vi "Test Clear Snapshot.vi"() -> (0 "error out":errorcluster)   [LabVIEW 2020]
doc: "Test Clearing Snapshot Entry of a single VI."
uses:
  <vilib>/addons/_JKI Toolkits/Caraya/classes/Test/Test.lvclass
  src/Public API.lvlib
  src/Path Getter Mock/Path Getter Mock.lvclass
  src/Type Definitions/Snapshot Handling Options--cluster.ctl
  C:/Users/juanj/Documents/hasbun_wood_engineering/github/Debug-Snapshots-for-LabVIEW/src/Path Getter Mock/Path Getter Mock.lvclass
  C:/Users/juanj/Documents/hasbun_wood_engineering/github/Debug-Snapshots-for-LabVIEW/src/IPath Getter/IPath Getter.lvclass
  <vilib>/Utility/miscctls.llb/LVBreakpointStatusEnum.ctl
  src/Type Definitions/Class Name--enum.ctl
  src/Type Definitions/Breakpoint--cluster.ctl
  src/Type Definitions/Debug Snapshot--cluster.ctl
  src/Type Definitions/Debug Snapshot Array--cluster.ctl
  <vilib>/addons/_JKI Toolkits/Caraya/classes/Assert/Assert.lvclass
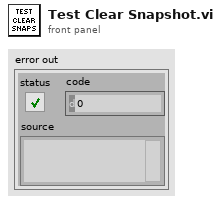
[diagram p1: front panel]
types:
  T1 = typedef "Debug Snapshot Array--cluster.ctl" = cluster{"Debug Snapshots":T2[]}
  T2 = typedef "Debug Snapshot--cluster.ctl" = cluster{"VI Name":string, "Breakpoints":T3[], "Probes":i32[]}
  T3 = typedef "Breakpoint--cluster.ctl" = cluster{"UID":i32, "BP Status":T4, "Class Name":T5}
  T4 = typedef "LVBreakpointStatusEnum.ctl" = enum8{"Cleared Break", "Enabled Break", "Disabled Break"}
  T5 = typedef "Class Name--enum.ctl" = enum16{"Node", "Wire"}
  T6 = typedef "Snapshot Handling Options--cluster.ctl" = cluster{"Breakpoints":bool, "Probes":bool}
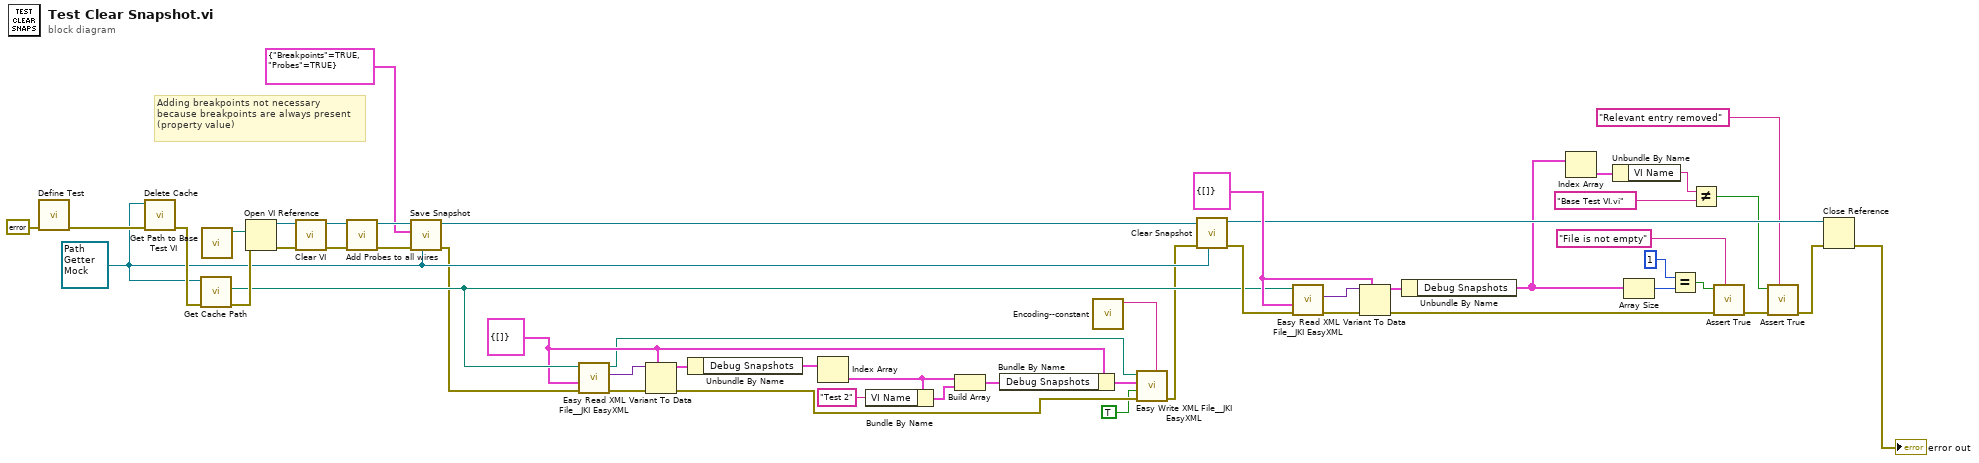
[diagram p0: block diagram]
diagram:
  w23 = T1 {"Debug Snapshots"=[]} ("Debug Snapshot Array")
  w37 = T1 {"Debug Snapshots"=[]} ("Debug Snapshot Array")
  w40 = refnum<class "Path Getter Mock.lvclass"> refnum ("Path Getter Mock.lvclass")
  # "Adding breakpoints not necessary\nbecause breakpoints are always present\n(property value)"
  n1 = call <vilib>:"Define Test.vi"("error in (no error)"=errorcluster {"status"=FALSE, "code"=0, "source"=""}) -> ("error out"=w49:errorcluster)  [unwired: 9 in, 1 out]
  n2 = call "Delete Cache.vi"("error in"=w49, "IPath Getter.lvclass"=w40) -> ("error out"=w46:errorcluster)  [unwired: 9 in]
  n3 = call-dynamic "Get Cache Path.vi"("error in"=w46, "Path Getter Mock in"=w40) -> ("error out"=w45:errorcluster, "Path"=w29:path)  [unwired: 8 in]
  n4 = call "Get Path to Base Test VI.vi"() -> ("Path"=w47:path)  [unwired: 11 in]
  n5 = Open VI Reference(vi path=w47, error in (no error)=w45) -> (vi reference=w2:refnum<vi>, error out=w48:errorcluster)  [unwired: 4 in]
  n6 = call "Clear VI.vi"("error in"=w48, "VI Refnum In"=w2) -> ("error out"=w3:errorcluster, "VI Refnum Out"=w1:refnum<vi>)  [unwired: 8 in]
  n7 = call "Add Probes to all wires.vi"("error in"=w3, "VI Refnum In"=w1) -> ("error out"=w43:errorcluster, "VI Refnum Out"=w44:refnum<vi>)  [unwired: 8 in]
  n8 = call "Save Snapshot.vi"("IPath Getter in"=w40, "error in"=w43, "Debug Elements Options"=T6 {"Breakpoints"=TRUE, "Probes"=TRUE}, "VI Reference in"=w44) -> ("error out"=w28:errorcluster, "VI Reference out"=w41:refnum<vi>)  [unwired: 6 in]
  n9 = call <vilib>:"Easy Read XML File__JKI EasyXML.vi"("error in (no error)"=w28, "LabVIEW Data (Type)"=w23, "XML File Path"=w29) -> ("error out"=w31:errorcluster, "LabVIEW Data"=w32:variant, "XML File Path (duplicate)"=w20:path)  [unwired: 6 in]
  n10 = Variant To Data(error in=w31, type=w23, Variant=w32) -> (data=w30:T1, error out=w19:errorcluster)
  n11 = Unbundle By Name(w30) -> ("Debug Snapshots"=w27:T2[])
  n12 = Index Array(array=w27) -> (element=w24:T2)  [unwired: 1 in]
  n13 = Bundle By Name(cluster=w24, "VI Name"="Test 2") -> (w25:T2)
  n14 = Build Array(w24, w25) -> (w22:T2[])
  n15 = Bundle By Name(cluster=w23, "Debug Snapshots"=w22) -> (w21:T1)
  n16 = call "Encoding--constant.vi"() -> ("Encoding (none)"=w18:string)  [unwired: 11 in]
  n17 = call <vilib>:"Easy Write XML File__JKI EasyXML.vi"("Encoding (none)"=w18, "error in (no error)"=w19, "Overwrite File? (false)"=TRUE, "LabVIEW Data"=w21, "XML File Path"=w20) -> ("error out"=w17:errorcluster)  [unwired: 5 in, 1 out]
  n18 = call "Clear Snapshot.vi"("IPath Getter.lvclass"=w40, "error in"=w17, "VI Reference in"=w41) -> ("error out"=w39:errorcluster, "VI Reference out"=w35:refnum<vi>)  [unwired: 7 in]
  n19 = call <vilib>:"Easy Read XML File__JKI EasyXML.vi"("error in (no error)"=w39, "LabVIEW Data (Type)"=w37, "XML File Path"=w29) -> ("error out"=w36:errorcluster, "LabVIEW Data"=w38:variant)  [unwired: 6 in, 1 out]
  n20 = Variant To Data(error in=w36, type=w37, Variant=w38) -> (data=w33:T1, error out=w34:errorcluster)
  n21 = Unbundle By Name(w33) -> ("Debug Snapshots"=w9:T2[])
  n22 = Index Array(array=w9) -> (element=w8:T2)  [unwired: 1 in]
  n23 = Unbundle By Name(w8) -> ("VI Name"=w10:string)
  n24 = Array Size(array=w9) -> (size(s)=w15:i32)
  n25 = Equal?(x=1, y=w15) -> (x = y?=w13:bool)
  n26 = Not Equal?(x=w10, y="Base Test VI.vi") -> (x != y?=w5:bool)
  n27 = call <vilib>:"Assert True.vi"("Label"="File is not empty", "error in (no error)"=w34, "True?"=w13) -> ("error out"=w7:errorcluster)  [unwired: 7 in, 1 out]
  n28 = call <vilib>:"Assert True.vi"("Label"="Relevant entry removed", "error in (no error)"=w7, "True?"=w5) -> ("error out"=w6:errorcluster)  [unwired: 7 in, 1 out]
  n29 = Close Reference(reference=w35, error in (no error)=w6) -> (error out=→"error out":errorcluster)
